vi "Lin_Rohner_lab4A_Compensation.vi"() -> ()   [LabVIEW 2019]
uses:
  <vilib>/Platform/TimedLoop/XDataNode/timing_clust.ctl
  <vilib>/Platform/TimedLoop/XDataNode/nitl_modes.ctl
  <vilib>/Platform/TimedLoop/XDataNode/wakeup.ctl
  <vilib>/Analysis/3filter.llb/Filter Passband Type.ctl
  <vilib>/DAQmx/write.llb/DAQmx Write (Analog DBL 1Chan 1Samp).vi
  <vilib>/DAQmx/read.llb/DAQmx Read (Analog DBL 1Chan 1Samp).vi
  <vilib>/DAQmx/create/channels.llb/DAQmx Create Channel (AO-Voltage-Basic).vi
  <vilib>/DAQmx/miscellaneous.llb/DAQmx Fill In Error Info.vi
  <vilib>/DAQmx/create/channels.llb/DAQmx Create Channel (AI-Voltage-Basic).vi
  <vilib>/platform/TimedLoop/XDataNode/XDataNode.xnode
  <vilib>/Platform/TimedLoop/XDataNode/XDNodeRunTimeDep.lvlib
  <vilib>/ptbypt/NI_PtbyPt.lvlib
  <vilib>/Analysis/NI_AALBase.lvlib
panel:
  out "Compensation Voltage":dbl
  out "Compensation Voltage":dbl(graph)
  out "Gravity Compesation":dbl
  out "Friction Compensation":dbl
  in  "Friction Compensation":bool
  out "Filtered Angular Velocity [rad/s]":dbl(graph)
  out "Filtered Angular Velocity [rad/s]":dbl
  in  "low cutoff freq:  Velocity":dbl=0.125 format="%0.3f"
  in  "Gravaty Compensation":bool
  out "Filtered Angular Position [rad]":dbl(graph)
  out "Filtered Angular Position [rad]":dbl
  out "Friction Compensation":dbl(graph)
  out "Gravity Compesation":dbl(graph)
  in  "low cutoff freq: Position":dbl=0.125 format="%0.3f"
  in  "stop":bool
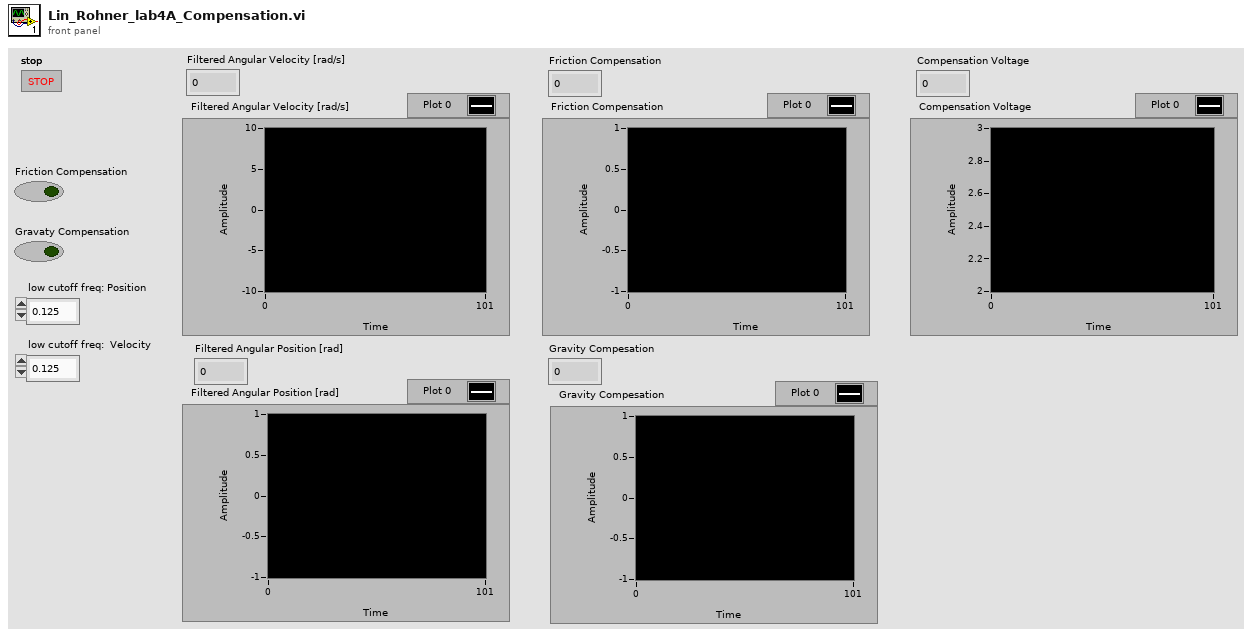
[diagram p1: front panel]
types:
  T1 = typedef "NI_AALBase.lvlib/Filter Passband Type.ctl" = enum32{"Lowpass", "Highpass", "Bandpass", "Bandstop"}
  T2 = typedef "XDNodeRunTimeDep.lvlib/timing_clust.ctl" = cluster{"Expected End [f-1]":u64, "Actual End [f-1]":u64, "Finished Late? [f-1]":bool, "Expected End [i-1]":u64, "Actual End [i-1]":u64, "Finished Late? [i-1]":bool, "Expected Start [i]":u64, "Actual Start [i]":u64, "Expected Start [f]":u64, "Actual Start [f]":u64, "Source Name":string, "Structure Name":string, "Period":i64, "Deadline":i64, "Offset":i64, "Start":i64, "Priority":i32, "Timeout":i32, "Mode":T3, "Wakeup Reason":T4, "Error":errorcluster, "Source Type":string, "Secondary Source Type":string, "Global End Time":u64, "Global Start Time":u64, "Frame Duration":u64, "Iteration Duration":u64, "Assigned CPU":i32, "I/O Scan Engine Mode":u32}
  T3 = typedef "XDNodeRunTimeDep.lvlib/nitl_modes.ctl" = enum32{"No Change", "Process missed periods, maintain original phase", "Discard missed periods, maintain original phase", "Process missed periods, ignore original phase", "Discard missed periods, ignore original phase"}
  T4 = typedef "XDNodeRunTimeDep.lvlib/wakeup.ctl" = enum32{"Normal", "Aborted", "Asynchronous wakeup", "Timing source error", "Timed loop error", "Timeout"}
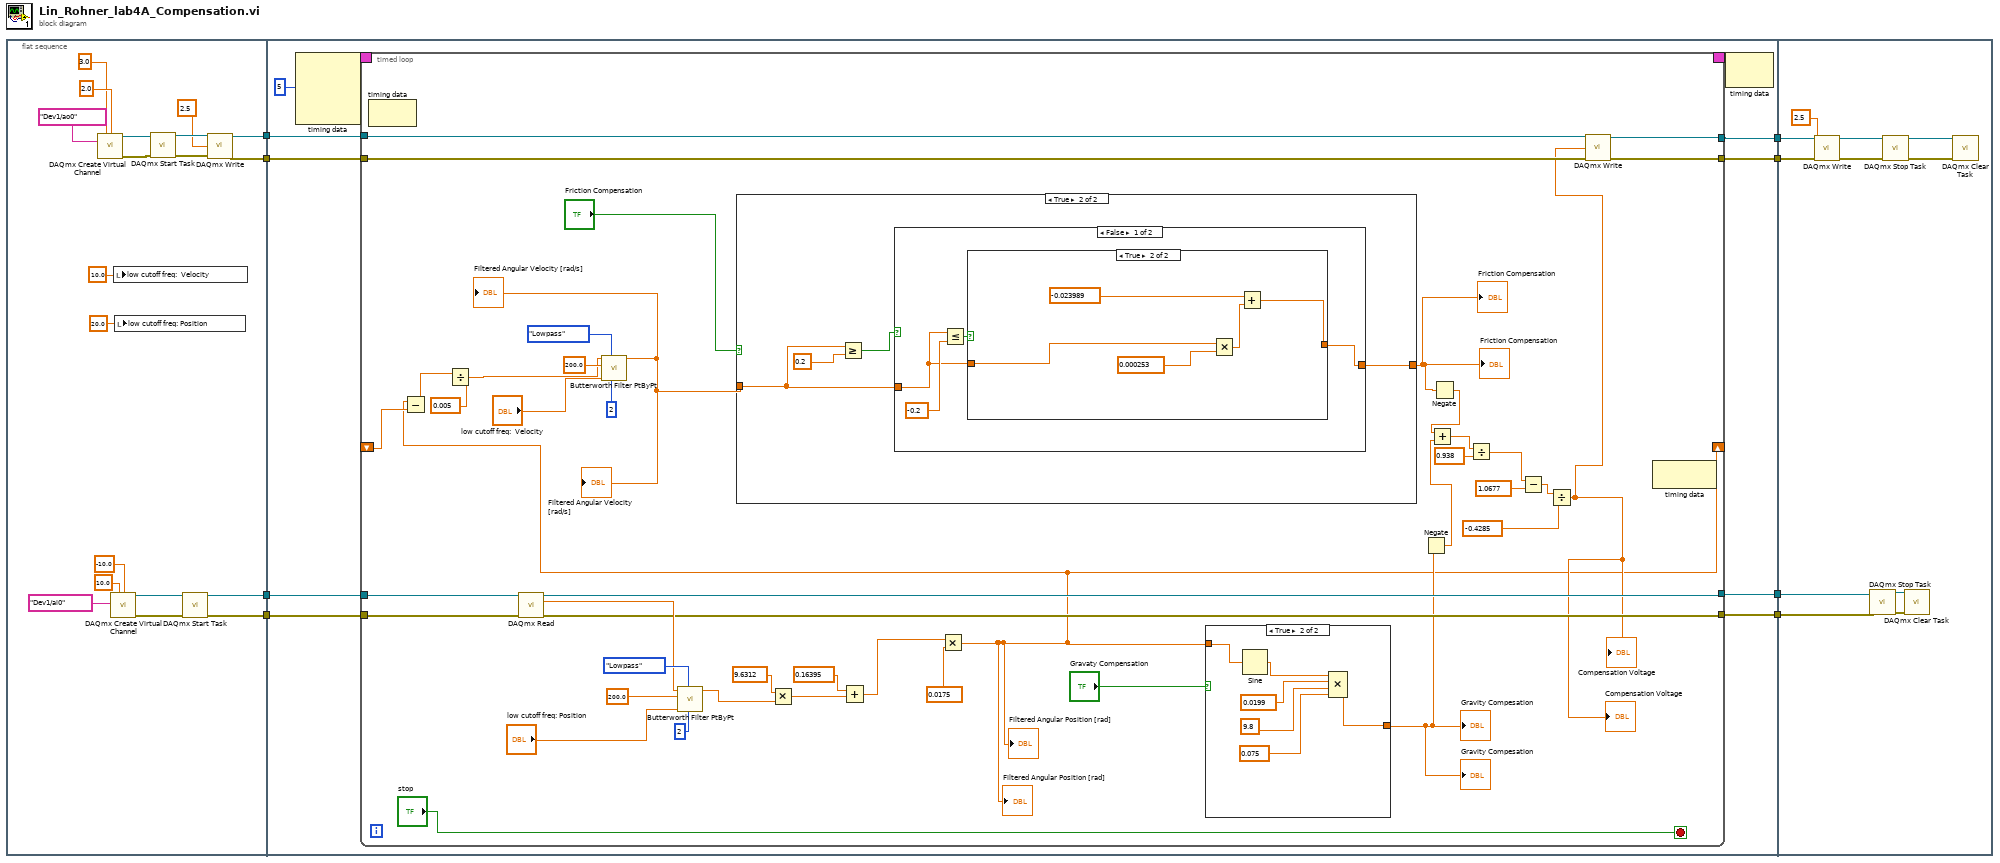
[diagram p0: block diagram]
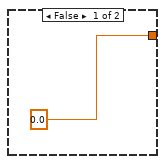
[diagram p2: hidden frame]
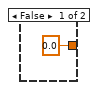
[diagram p3: hidden frame]
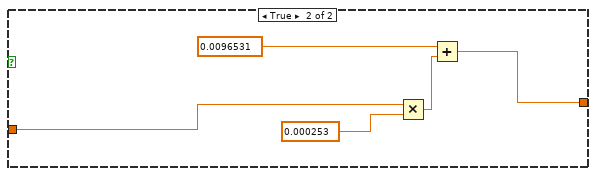
[diagram p4: hidden frame]
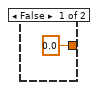
[diagram p5: hidden frame]
diagram:
  n1 = flat-sequence {
    tunnel: [w25] -> w8
    tunnel: [w24] -> w7
    tunnel: [w13] -> w6
    tunnel: [w12] -> w5
    tunnel: w8 -> [w35]
    tunnel: w7 -> [w34]
    tunnel: w6 -> [w33]
    tunnel: w5 -> [w32]
    tunnel: [w31] -> w4
    tunnel: [w30] -> w3
    tunnel: [w29] -> w2
    tunnel: [w28] -> w1
    tunnel: w4 -> [w118]
    tunnel: w3 -> [w117]
    tunnel: w2 -> [w116]
    tunnel: w1 -> [w115]
    frame #0 {
      n2 = call-poly <vilib>:"DAQmx Create Virtual Channel.vi"("maximum value"=3.0, "minimum value"=2.0, "physical channels"=tag "Dev1/ao0") -> ("task out"=w27:refnum<k21>, "error out"=w23:errorcluster)  [unwired: 11 in]
      n3 = call-poly <vilib>:"DAQmx Create Virtual Channel.vi"("maximum value"=10.0, "minimum value"=-10.0, "physical channels"=tag "Dev1/ai0") -> ("task out"=w14:refnum<k21>, "error out"=w15:errorcluster)  [unwired: 11 in]
      n4 = local write "low cutoff freq:  Velocity"(10.0 ("low cutoff freq:  Velocity")) -> ()
      n5 = local write "low cutoff freq: Position"(20.0 ("low cutoff freq: Position")) -> ()
      n6 = call <vilib>:"DAQmx Start Task.vi"("task/channels in"=w27, "error in"=w23) -> ("task out"=w26:refnum<k21>, "error out"=w22:errorcluster)  [unwired: 12 in]
      n7 = call <vilib>:"DAQmx Start Task.vi"("task/channels in"=w14, "error in"=w15) -> ("task out"=w13:refnum<k21>, "error out"=w12:errorcluster)  [unwired: 12 in]
      n8 = call-poly <vilib>:"DAQmx Write.vi"("task/channels in"=w26, "data"=2.5, "error in"=w22) -> ("task out"=w25:refnum<k21>, "error out"=w24:errorcluster)  [unwired: 10 in, 1 out]
    }
    frame #1 {
      n9 = node-c288(i64 5 ("Period")) -> (w38:T2)  [unwired: 3 in]
      n10 = timed-loop {
        timing: w38 -> [_]
        timing-out: [_] -> w37
        tunnel: w35 -> [w73]
        tunnel: w34 -> [w72]
        tunnel: w33 -> [w71]
        tunnel: w32 -> [w70]
        tunnel: [w66] -> w31
        tunnel: [w65] -> w30
        tunnel: [w69] -> w29
        tunnel: [w68] -> w28
        shift-right: [w41] -> _
        shift-left: _ -> [w54]
        stop <- "stop" stop-if-true
        n11 = node-c288() -> ()  [unwired: 1 in, 1 out]
        n12 = call-poly <vilib>:"DAQmx Read.vi"("task/channels in"=w71, "error in"=w70) -> ("task out"=w69:refnum<k21>, "data"=w74:dbl, "error out"=w68:errorcluster)  [unwired: 11 in]
        n13 = call <vilib>:"Butterworth Filter PtByPt.vi"("order"=2, "filter type"=Filter_Passband_Type."Lowpass", "low cutoff freq: fl"="low cutoff freq: Position", "sampling freq: fs"=200.0, "x"=w74) -> ("Filtered x"=w75:dbl)  [unwired: 4 in, 1 out]
        n14 = Multiply(x=9.6312, y=w75) -> (x*y=w77:dbl)
        n15 = Add(x=0.16395, y=w77) -> (x+y=w63:dbl)
        n16 = Multiply(x=w63, y=0.0175) -> (x*y=w41:dbl)
        "Filtered Angular Position [rad]" <- w41
        "Filtered Angular Position [rad]" <- w41
        n17 = Subtract(x=w41, y=w54) -> (x-y=w61:dbl)
        n18 = Divide(x=w61, y=0.005) -> (x/y=w56:dbl)
        n19 = call <vilib>:"Butterworth Filter PtByPt.vi"("order"=2, "filter type"=Filter_Passband_Type."Lowpass", "low cutoff freq: fl"="low cutoff freq:  Velocity", "sampling freq: fs"=200.0, "x"=w56) -> ("Filtered x"=w53:dbl)  [unwired: 4 in, 1 out]
        "Filtered Angular Velocity [rad/s]" <- w53
        "Filtered Angular Velocity [rad/s]" <- w53
        n20 = case shown="True" "Friction Compensation" {
          tunnel: [0.0 ("f") w84] -> w40
          tunnel: w53 -> [_ w85]
          frame False {
          }
          frame True {
            n21 = Greater Or Equal?(x=w85, y=0.2) -> (x >= y?=w83:bool)
            n22 = case shown="False" w83 {
              tunnel: w85 -> [w88 w98]
              tunnel: [w87 w99] -> w84
              frame False {
                n23 = Less Or Equal?(x=w88, y=-0.2) -> (x <= y?=w89:bool)
                n24 = case shown="True" w89 {
                  tunnel: w88 -> [_ w94]
                  tunnel: [0.0 w93] -> w87
                  frame False {
                  }
                  frame True {
                    n25 = Multiply(x=w94, y=0.000253) -> (x*y=w95:dbl)
                    n26 = Add(x=-0.023989, y=w95) -> (x+y=w93:dbl)
                  }
                }
              }
              frame True {
                n27 = Multiply(x=w98, y=0.000253) -> (x*y=w100:dbl)
                n28 = Add(x=0.0096531, y=w100) -> (x+y=w99:dbl)
              }
            }
          }
        }
        "Friction Compensation" <- w40
        "Friction Compensation" <- w40
        n29 = case shown="True" "Gravaty Compensation" {
          tunnel: [0.0 w104] -> w43
          tunnel: w41 -> [_ w103]
          frame False {
          }
          frame True {
            n30 = Sine(x=w103) -> (sin(x)=w108:dbl)
            n31 = Compound Arithmetic op=MULTIPLY(w108, 0.0199 ("y"), 9.8 ("value"), 0.075 ("value")) -> (w104:dbl)
          }
        }
        "Gravity Compesation" <- w43
        "Gravity Compesation" <- w43
        n32 = Negate(x=w43) -> (-x=w42:dbl)
        n33 = Negate(x=w40) -> (-x=w39:dbl)
        n34 = Add(x=w39, y=w42) -> (x+y=w51:dbl)
        n35 = Divide(x=w51, y=0.938) -> (x/y=w48:dbl)
        n36 = Subtract(x=w48, y=1.0677) -> (x-y=w46:dbl)
        n37 = Divide(x=w46, y=-0.4285) -> (x/y=w44:dbl)
        "Compensation Voltage" <- w44
        "Compensation Voltage" <- w44
        n38 = call-poly <vilib>:"DAQmx Write.vi"("task/channels in"=w73, "data"=w44, "error in"=w72) -> ("task out"=w66:refnum<k21>, "error out"=w65:errorcluster)  [unwired: 10 in, 1 out]
        n39 = node-c288() -> ()  [unwired: 1 in, 1 out]
      }
      n40 = node-c288(w37) -> ()  [unwired: 1 out]
    }
    frame #2 {
      n41 = call-poly <vilib>:"DAQmx Write.vi"("task/channels in"=w118, "data"=2.5, "error in"=w117) -> ("task out"=w125:refnum<k21>, "error out"=w122:errorcluster)  [unwired: 10 in, 1 out]
      n42 = call <vilib>:"DAQmx Stop Task.vi"("task/channels in"=w116, "error in"=w115) -> ("task out"=w119:refnum<k21>, "error out"=w120:errorcluster)  [unwired: 12 in]
      n43 = call <vilib>:"DAQmx Stop Task.vi"("task/channels in"=w125, "error in"=w122) -> ("task out"=w124:refnum<k21>, "error out"=w123:errorcluster)  [unwired: 12 in]
      n44 = call <vilib>:"DAQmx Clear Task.vi"("task in"=w119, "error in"=w120) -> ()  [unwired: 13 in, 1 out]
      n45 = call <vilib>:"DAQmx Clear Task.vi"("task in"=w124, "error in"=w123) -> ()  [unwired: 13 in, 1 out]
    }
  }
